vi "subFixUpLooseFiles.vi"(8 "error in (no error)":errorcluster, 9 "Loose files":path[](array[path])=[path "E:/Repos/LVDependencyInspector/obj/DependencyInspector.vi"], 10 "Dependency order":T1[](array[typedef])=[{"Library ref"=refnum, "Target path"=path "E:/Repos/LVDependencyInspector/obj/Addons/LabVIEWObjectInterfaces.lvlibp", "Source name"="LabVIEWObjectInterfaces.lvlib", "Build spec name"="LabVIEWObjectInterfaces"}, {"Library ref"=refnum, "Target path"=path "E:/Repos/LVDependencyInspector/obj/Addons/ErrorManager.lvlibp", "Source name"="ErrorManager.lvlib", "Build spec name"="ErrorManager"}, {"Library ref"=refnum, "Target path"=path "E:/Repos/LVDependencyInspector/obj/Addons/ExtensionInterfaces.lvlibp", "Source name"="ExtensionInterfaces.lvlib", "Build spec name"="ExtensionInterfaces"}, {"Library ref"=refnum, "Target path"=path "E:/Repos/LVDependencyInspector/obj/Addons/LabVIEWItem.lvlibp", "Source name"="LabVIEWItem.lvlib", "Build spec name"="LabVIEWItem"}, {"Library ref"=refnum, "Target path"=path "E:/Repos/LVDependencyInspector/obj/Addons/DefaultExtensions.lvlibp", "Source name"="DefaultExtensions.lvlib", "Build spec name"="DefaultExtensions"}, {"Library ref"=refnum, "Target path"=path "E:/Repos/LVDependencyInspector/obj/Addons/LabVIEWContainers.lvlibp", "Source name"="LabVIEWContainers.lvlib", "Build spec name"="LabVIEWContainers"}, {"Library ref"=refnum, "Target path"=path "E:/Repos/LVDependencyInspector/obj/Addons/LabVIEWFiles.lvlibp", "Source name"="LabVIEWFiles.lvlib", "Build spec name"="LabVIEWFiles"}, {"Library ref"=refnum, "Target path"=path "E:/Repos/LVDependencyInspector/obj/Addons/LabVIEWObjectFactory.lvlibp", "Source name"="LabVIEWObjectFactory.lvlib", "Build spec name"="LabVIEWObjectFactory"}, {"Library ref"=refnum, "Target path"=path "E:/Repos/LVDependencyInspector/obj/Addons/DependencyInspection.lvlibp", "Source name"="DependencyInspection.lvlib", "Build spec name"="DependencyInspection"}, {"Library ref"=refnum, "Target path"=path "E:/Repos/LVDependencyInspector/obj/Addons/DependencyInspector.lvlibp", "Source name"="DependencyInspector.lvlib", "Build spec name"="DependencyInspector"}, {"Library ref"=refnum, "Target path"=path "", "Source name"="Application", "Build spec name"="Application"}], 11 "Local Host App Instance":refnum<vi>) -> (0 "error out":errorcluster)   [LabVIEW 2020, in "SolutionBuilder.lvlib"]
uses:
  SolutionBuilder.lvlib
  FileInfo.ctl
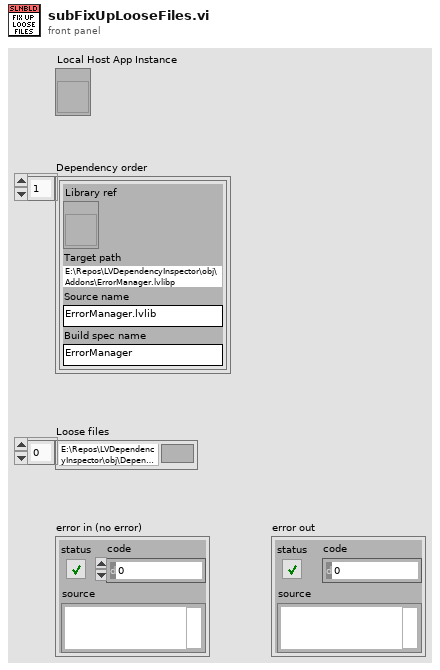
[diagram p1: front panel]
types:
  T1 = typedef "SolutionBuilder.lvlib/FileInfo.ctl" = cluster{"Library ref":refnum<vi>, "Target path":path, "Source name":string, "Build spec name":string}
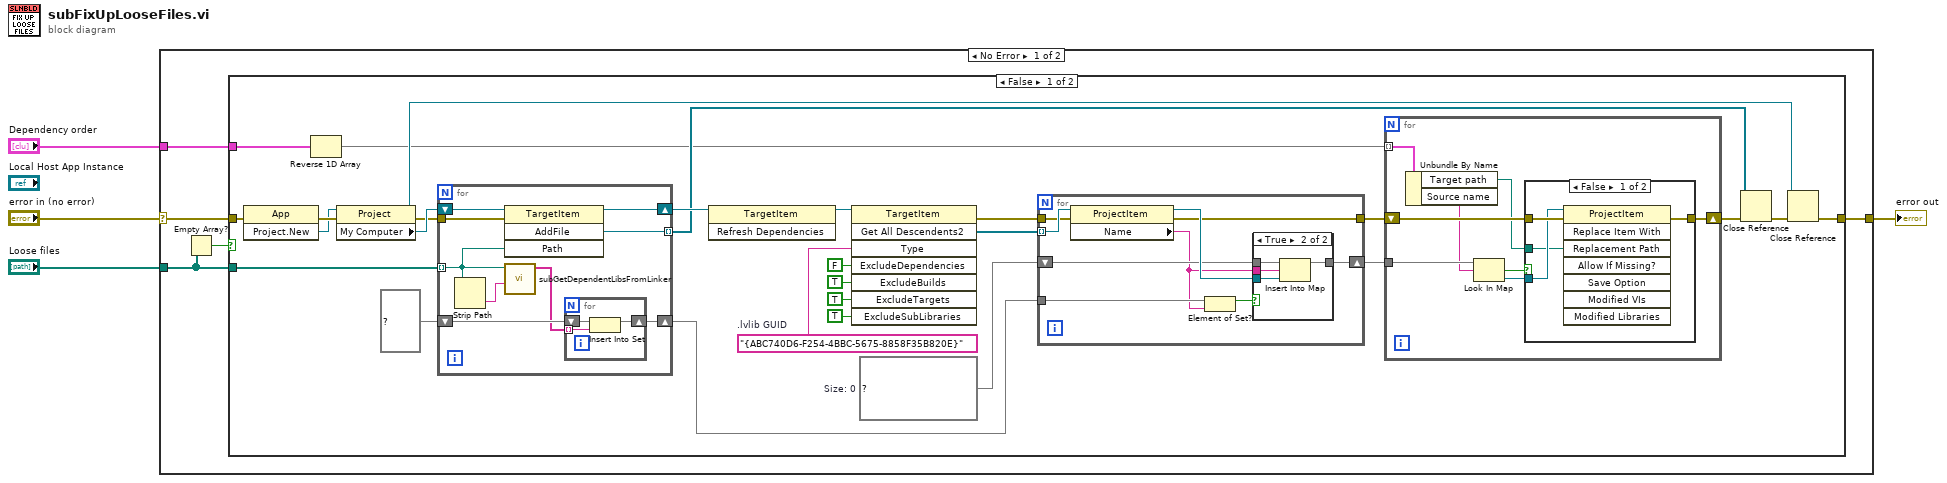
[diagram p0: block diagram]
diagram:
  n1 = case shown="No Error" "error in (no error)" {
    selector: "error in (no error)" -> [w7 w77]
    tunnel: "Loose files" -> [w6 _]
    tunnel: "Dependency order" -> [w9 _]
    tunnel: [w8 w77] -> w2
    frame No Error {
      n2 = Empty Array?(array=w6) -> (empty?=w5:bool)
      n3 = case shown="False" w5 {
        tunnel: w6 -> [w36 _]
        tunnel: w9 -> [w35 _]
        tunnel: [w34 w76] -> w8
        tunnel: w7 -> [w10 w76]
        frame False {
          w14 = map{string, refnum<vi>} {}  # Size: 0
          w22 = "{ABC740D6-F254-4BBC-5675-8858F35B820E}"  # .lvlib GUID
          n4 = invoke class="App" method="Project.New"(error in=w10) -> (error out=w32:errorcluster, "Project:New"=w26:refnum<vi>)  [unwired: 2 in, 1 out]
          n5 = Reverse 1D Array(array=w35) -> (reversed array=w24:T1[])
          n6 = property class="Project"(reference=w26, error in=w32) -> (reference out=w29:refnum<vi>, error out=w31:errorcluster, "My Computer"=w33:refnum<vi>)
          n7 = for {
            tunnel: w31 -> [w44]
            tunnel: w36 -> [w41] mode=indexing
            tunnel: [w43] -> w27 mode=indexing
            shift-right: [w42] -> w28
            shift-left: w33 -> [w45]
            shift-right: [w39] -> w11
            shift-left: set{string} {} ("set in") -> [w38]
            n8 = Strip Path(path=w41) -> (name=w40:string)  [unwired: 1 out]
            n9 = invoke class="TargetItem" method="AddFile"(reference=w45, error in=w44, "Path"=w41) -> (reference out=w42:refnum<vi>, "AddFile"=w43:refnum<vi>)  [unwired: 1 in, 2 out]
            n10 = call "subGetDependentLibsFromLinker.vi"("Name"=w40, "Path"=w41) -> ("Dependent libs"=w37:string[])  [unwired: 9 in]
            n11 = for {
              shift-right: [w48] -> w39
              shift-left: w38 -> [w47]
              tunnel: w37 -> [w46] mode=indexing
              n12 = Insert Into Set(10:w46, 11:w47) -> (3:w48:set{string})  [unwired: 1 out]
            }
          }
          n13 = invoke class="TargetItem" method="Refresh Dependencies"(reference=w28) -> (reference out=w17:refnum<vi>)  [unwired: 2 in, 2 out]
          n14 = invoke class="TargetItem" method="Get All Descendents2"(reference=w17, "Type"=w22, "ExcludeDependencies"=FALSE, "ExcludeBuilds"=TRUE, "ExcludeTargets"=TRUE, "ExcludeSubLibraries"=TRUE) -> (error out=w16:errorcluster, "Get All Descendents2"=w15:refnum<vi>[])  [unwired: 2 in, 6 out]
          n15 = for {
            tunnel: w15 -> [w57] mode=indexing
            tunnel: w16 -> [w56]
            shift-right: [w54] -> w13
            shift-left: w14 -> [w53]
            tunnel: [w52] -> w12
            tunnel: w11 -> [w51]
            n16 = property class="ProjectItem"(reference=w57, error in=w56) -> (reference out=w55:refnum<vi>, error out=w52:errorcluster, "Name"=w50:string)
            n17 = Element of Set?(10:w50, 11:w51) -> (3:w49:bool)
            n18 = case shown="True" w49 {
              tunnel: w55 -> [_ w62]
              tunnel: [w58 w61] -> w54
              tunnel: w53 -> [w58 w60]
              tunnel: w50 -> [_ w59]
              frame False {
              }
              frame True {
                n19 = Insert Into Map(map in=w60, key=w59, value=w62) -> (map out=w61:map{string, refnum<vi>})  [unwired: 2 out]
              }
            }
          }
          n20 = for {
            tunnel: w13 -> [w70]
            tunnel: w24 -> [w67] mode=indexing
            shift-right: [w68] -> w25
            shift-left: w12 -> [w69]
            n21 = Unbundle By Name(w67) -> ("Target path"=w63:path, "Source name"=w66:string)
            n22 = Look In Map(map=w70, key=w66) -> (key not found?=w65:bool, value=w64:refnum<vi>)  [unwired: 1 in]
            n23 = case shown="False" w65 {
              tunnel: w69 -> [w74 w75]
              tunnel: [w73 w75] -> w68
              tunnel: w64 -> [w72 _]
              tunnel: w63 -> [w71 _]
              frame False {
                n24 = invoke class="ProjectItem" method="Replace Item With"(reference=w72, error in=w74, "Replacement Path"=w71) -> (error out=w73:errorcluster)  [unwired: 5 in, 7 out]
              }
              frame True {
              }
            }
          }
          n25 = Close Reference(reference=w27, error in (no error)=w25) -> (error out=w30:errorcluster)
          n26 = Close Reference(reference=w29, error in (no error)=w30) -> (error out=w34:errorcluster)
        }
        frame True {
        }
      }
    }
    frame Error {
    }
  }
  "error out" <- w2
